vi "_FPGA_wfmMUX.vi"(0 "OppAux":fxp<+/-,16,14>, 1 "Aux":fxp<+/-,16,14>, 2 "Sel":u8, 5 "OppPri":fxp<+/-,16,14>, 7 "Pri+Aux":fxp<+/-,16,14>, 9 "OppPri+OppAux":fxp<+/-,16,14>, 11 "FGEN":fxp<+/-,16,14>, 12 "Pri+OppAux":fxp<+/-,16,14>, 13 "OppPri+Aux":fxp<+/-,16,14>, 14 "Pri":fxp<+/-,16,14>) -> (4 "SelectedWfm":fxp<+/-,16,14>)   [LabVIEW 2018]
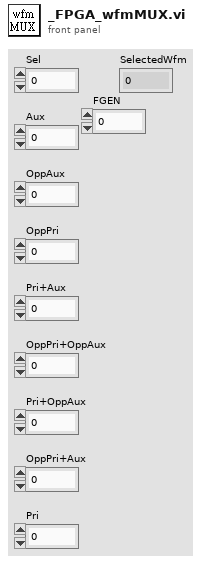
[diagram p1: front panel]
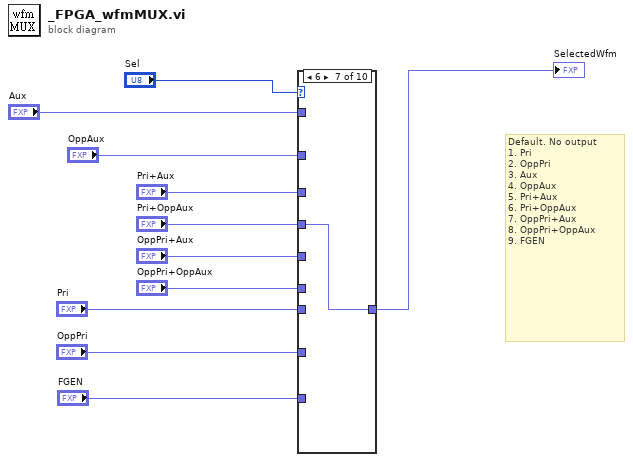
[diagram p0: block diagram]
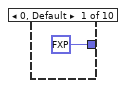
[diagram p2: hidden frame]
diagram:
  # "Default. No output\n1. Pri\n2. OppPri\n3. Aux\n4. OppAux\n5. Pri+Aux\n6. Pri+OppAux\n7. OppPri+Aux\n8. OppPri+OppAux\n9. FGEN"
  n1 = case shown="6" "Sel" {
    tunnel: "Aux" -> [_ _ _ w15 _ _ _ _ _ _]
    tunnel: "OppAux" -> [_ _ _ _ w16 _ _ _ _ _]
    tunnel: "Pri+Aux" -> [_ _ _ _ _ w17 _ _ _ _]
    tunnel: "Pri+OppAux" -> [_ _ _ _ _ _ w18 _ _ _]
    tunnel: "OppPri+Aux" -> [_ _ _ _ _ _ _ w19 _ _]
    tunnel: "OppPri+OppAux" -> [_ _ _ _ _ _ _ _ w20 _]
    tunnel: "Pri" -> [_ w13 _ _ _ _ _ _ _ _]
    tunnel: "OppPri" -> [_ _ w14 _ _ _ _ _ _ _]
    tunnel: [fxp<+/-,16,14> 0.0 ("OppPri+OppAux") w13 w14 w15 w16 w17 w18 w19 w20 w21] -> w11
    tunnel: "FGEN" -> [_ _ _ _ _ _ _ _ _ w21]
    frame 0, Default {
    }
    frame 1 {
    }
    frame 2 {
    }
    frame 3 {
    }
    frame 4 {
    }
    frame 5 {
    }
    frame 6 {
    }
    frame 7 {
    }
    frame 8 {
    }
    frame 9 {
    }
  }
  "SelectedWfm" <- w11
